vi "Create Calibration Point Check.vi"(8 "error in (no error)":errorcluster, 9 "Reset?":bool, 10 "Pass Flag?":bool, 11 "Steady State Duration":i32) -> (0 "error out":errorcluster, 3 "Record?":bool)   [LabVIEW 2026, in "Processing_Engine.lvlib"]
uses:
  Processing_Engine.lvlib
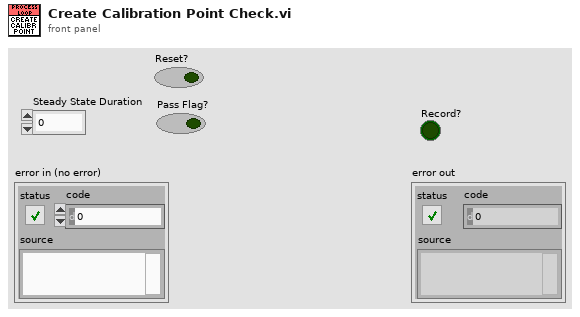
[diagram p1: front panel]
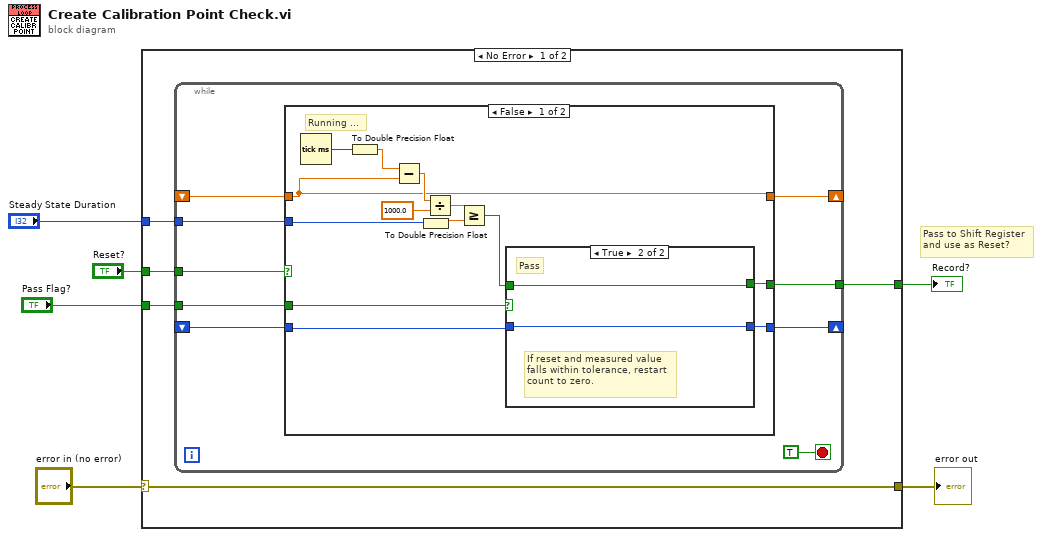
[diagram p0: block diagram]
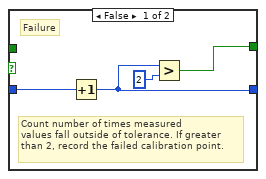
[diagram p2: hidden frame]
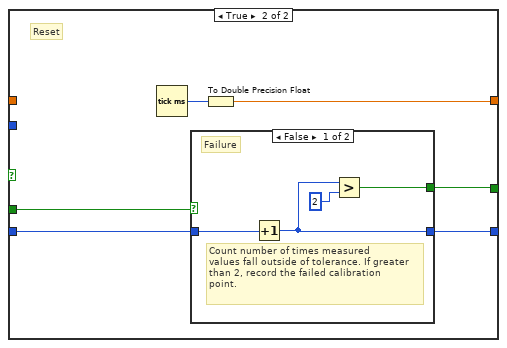
[diagram p3: hidden frame]
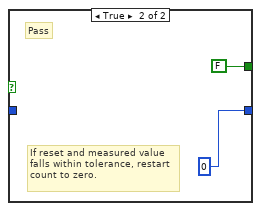
[diagram p4: hidden frame]
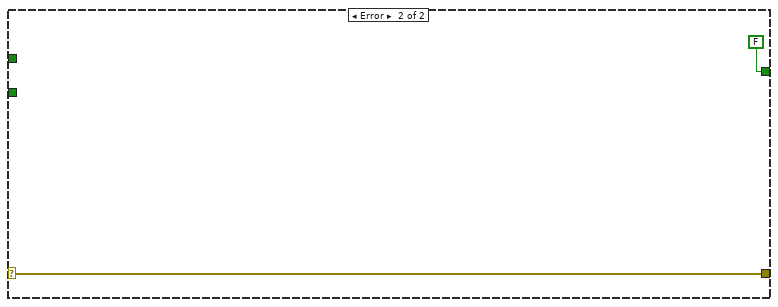
[diagram p5: hidden frame]
diagram:
  # "Pass to Shift Register\nand use as Reset?"
  n1 = case shown="No Error" "error in (no error)" {
    selector: "error in (no error)" -> [w8 w53]
    tunnel: "Steady State Duration" -> [w11 _]
    tunnel: "Pass Flag?" -> [w10 _]
    tunnel: [w9 FALSE] -> w4
    tunnel: [w8 w53] -> w2
    tunnel: "Reset?" -> [w7 _]
    frame No Error {
      n2 = while {
        tunnel: w11 -> [w17]
        tunnel: w10 -> [w12]
        shift-right: [w19] -> _
        shift-left: _ -> [w18]
        tunnel: [w16] -> w9
        shift-right: [w15] -> _
        shift-left: _ -> [w14]
        tunnel: w7 -> [w13]
        stop <- TRUE stop-if-true
        n3 = case shown="False" w13 {
          tunnel: [w26 w44] -> w19
          tunnel: w18 -> [w26 _]
          tunnel: w17 -> [w31 _]
          tunnel: [w22 w40] -> w16
          tunnel: [w21 w41] -> w15
          tunnel: w12 -> [w25 w43]
          tunnel: w14 -> [w24 w42]
          frame False {
            # "Running ..."
            n4 = Tick Count (ms)() -> (millisecond timer value=w28:u32)
            n5 = To Double Precision Float(number=w28) -> (double precision float=w27:dbl)
            n6 = Subtract(x=w27, y=w26) -> (x-y=w29:dbl)
            n7 = To Double Precision Float(number=w31) -> (double precision float=w30:dbl)
            n8 = Divide(x=w29, y=1000.0) -> (x/y=w32:dbl)
            n9 = Greater Or Equal?(x=w32, y=w30) -> (x >= y?=w23:bool)
            n10 = case shown="True" w25 {
              tunnel: w24 -> [w37 w39]
              tunnel: [w36 w39] -> w21
              tunnel: [w34 w38] -> w22
              tunnel: w23 -> [_ w38]
              frame False {
                # "Failure"
                # "Count number of times measured \nvalues fall outside of tolerance. If greater\nthan 2, record the failed calibration point."
                n11 = Increment(x=w37) -> (x+1=w36:i32)
                n12 = Greater?(x=w36, y=2) -> (0:w34:bool)
              }
              frame True {
                # "Pass"
                # "If reset and measured value\nfalls within tolerance, restart\ncount to zero."
              }
            }
          }
          frame True {
            # "Reset"
            n13 = Tick Count (ms)() -> (millisecond timer value=w45:u32)
            n14 = case shown="False" w43 {
              tunnel: w42 -> [w49 _]
              tunnel: [w48 0] -> w41
              tunnel: [w46 FALSE] -> w40
              frame False {
                # "Failure"
                # "Count number of times measured \nvalues fall outside of tolerance. If greater\nthan 2, record the failed calibration\npoint."
                n15 = Increment(x=w49) -> (x+1=w48:i32)
                n16 = Greater?(x=w48, y=2) -> (0:w46:bool)
              }
              frame True {
                # "Pass"
                # "If reset and measured value\nfalls within tolerance, restart\ncount to zero."
              }
            }
            n17 = To Double Precision Float(number=w45) -> (double precision float=w44:dbl)
          }
        }
      }
    }
    frame Error {
    }
  }
  "Record?" <- w4
  "error out" <- w2
